vi "ReloadConfigurationFile.vi"(8 "error in (no error)":errorcluster, 10 "reference In":refnum<class "ModuleAdmin.lvclass">, 11 "ModuleID":i32) -> (0 "error out":errorcluster)   [LabVIEW 2018, in "AcPwrPlugins.lvlib" / "AcPwrBase.lvclass"]
uses:
  AcPwrBase.lvclass
  <userlib>/NIST/ModuleAdminLib/ModuleAdmin/ModuleAdmin.lvclass
  AcPwrModule/Protected/clEventType.ctl
  AcPwrModule/PublicAPI/Arguments/Broadcasts/clDidInit.ctl
  <vilib>/Utility/error.llb/Error Cluster From Error Code.vi
  <vilib>/ErrorRing/Error Ring.xnode
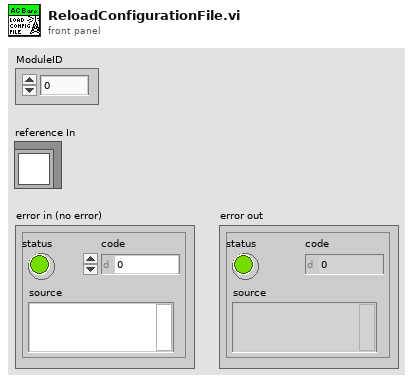
[diagram p1: front panel]
types:
  T1 = typedef "clBroadcastEvents.ctl" = cluster{"DidInit":refnum<user-event>, "StatusUpdate":refnum<user-event>, "ErrorReport":refnum<user-event>, "DidStop":refnum<user-event>, "PathToINI":refnum<user-event>, "Measurements":refnum<user-event>, "LoadConfigFile":refnum<user-event>, "GetSettings":refnum<user-event>, "SetSettings":refnum<user-event>, "GetType&ID":refnum<user-event>, "GotSettings":refnum<user-event>}
  T2 = typedef "clDidInit.ctl" = cluster{"Init?":bool, "ModuleAdmin":refnum<class "ModuleAdmin.lvclass">}
  T3 = typedef "clEventType.ctl" = cluster{"ModuleID":i32, "Data":variant}
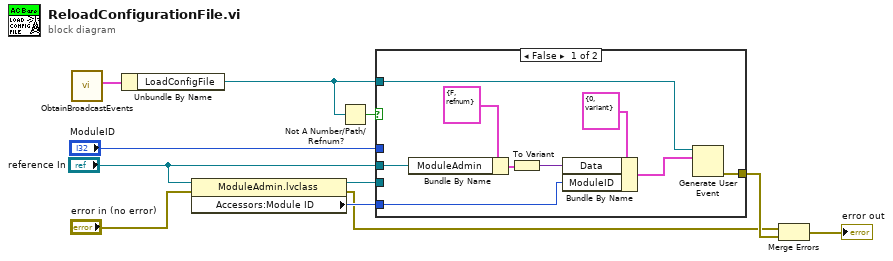
[diagram p0: block diagram]
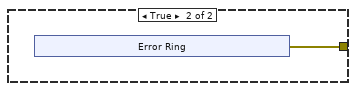
[diagram p2: hidden frame]
diagram:
  n1 = call "ObtainBroadcastEvents.vi"() -> ("clAcPwrEvents"=w11:T1)  [unwired: 10 in, 1 out]
  n2 = Unbundle By Name(w11) -> ("LoadConfigFile"=w7:refnum<user-event>)
  n3 = property class="ModuleAdmin.lvclass"(reference="reference In", error in="error in (no error)") -> (reference out=w3:refnum<class "ModuleAdmin.lvclass">, error out=w1:errorcluster, "Accessors:Module ID"=w2:i32)
  n4 = Not A Number/Path/Refnum?(number/path/refnum=w7) -> (NaN/Path/Refnum?=w8:bool)
  n5 = case shown="False" w8 {
    tunnel: "ModuleID" -> [_ _]
    tunnel: w7 -> [w18 _]
    tunnel: [w17 w21] -> w6
    tunnel: "reference In" -> [w14 _]
    tunnel: w3 -> [_ _]
    tunnel: w2 -> [w12 _]
    frame False {
      n6 = Bundle By Name(cluster=T2 {"Init?"=FALSE, "ModuleAdmin"=refnum} ("clDidInit"), "ModuleAdmin"=w14) -> (w13:T2)
      n7 = To Variant(anything=w13) -> (Variant=w16:variant)
      n8 = Bundle By Name(cluster=T3 {"ModuleID"=0, "Data"=variant} ("clEventType"), "Data"=w16, "ModuleID"=w12) -> (w19:T3)
      n9 = Generate User Event(user event=w18, event data cluster=w19) -> (error out=w17:errorcluster)  [unwired: 2 in, 1 out]
    }
    frame True {
      n10 = xnode "Error Ring"() -> ("error out"=w21:errorcluster)
    }
  }
  n11 = Merge Errors(w1, w6) -> (→"error out":errorcluster)
